vi "Do.vi"(8 "error in":errorcluster, 10 "Actor in":refnum<class "Actor.lvclass">, 11 "Stop MSG":refnum<class "Stop MSG.lvclass">) -> (0 "error out":errorcluster, 2 "Actor out":refnum<class "Actor.lvclass">)   [LabVIEW 2017, in "Controller.lvlib" / "Stop MSG.lvclass"]
doc: "(<B>Filename</B>: Actor Framework.lvlib:Message.lvclass:Do.vi)\n\nDefines what a message does when it is received by an actor. Generally, a message instructs an actor to invoke one of its methods. By default, this method does nothing. A child class must override it to define behavior. Create a child class by using the Actor Framework Message Maker dialog box."
uses:
  Stop MSG.lvclass
  <vilib>/ActorFramework/Actor/Actor.lvclass
  <vilib>/MSR Consulting, LLC/General Reuse/SuperActor/SuperActor.lvclass
  C:/Program Files (x86)/National Instruments/LabVIEW 2017/vi.lib/ActorFramework/Actor/Actor.lvclass
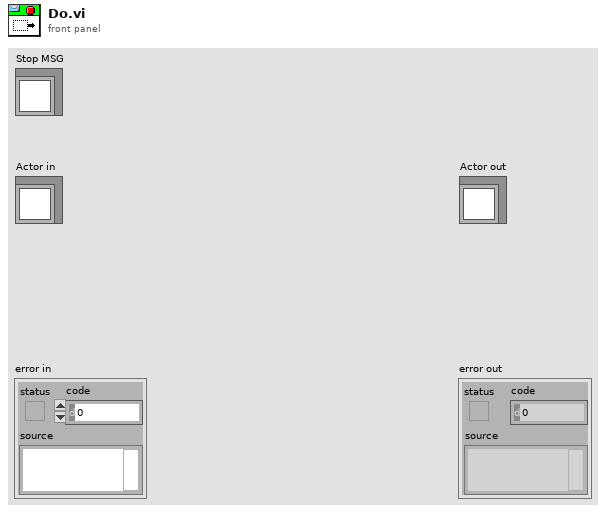
[diagram p1: front panel]
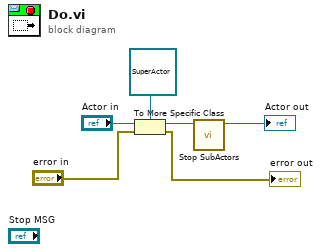
[diagram p0: block diagram]
diagram:
  n1 = To More Specific Class(target class=refnum<class "SuperActor.lvclass"> refnum ("SuperActor.lvlib:SuperActor"), reference="Actor in", error in="error in") -> (specific class reference=w4:refnum<class "SuperActor.lvclass">, error out=→"error out":errorcluster)
  n2 = call <vilib>:"Stop SubActors.vi"("SuperActor in"=w4) -> ("SuperActor out"=→"Actor out":refnum<class "SuperActor.lvclass">)  [unwired: 10 in]
